vi "水质测量数据table定义.vi"(5 "数据标记表":string(combo)="N", 7 "table 输入":string, 9 "SN":string, 10 "测量模式":T2(ring)=enum."水样测试", 11 "data":T1 {"单位" items=["ug/L", "mg/L", "ppm", "mg/m3", "cm", "ppb", "ug/m3", "%", "nmol/mol", "umol/mol", "MPN/L", "MPN/100ml", "ng/m3", "NTU", "无量纲", "ms/cm", "us/cm"]}) -> (1 "table 输出":string, 2 "columns":string[](array[string]), 3 "data输出":T3)   [LabVIEW 2016, in "挥发酚.lvlib"]
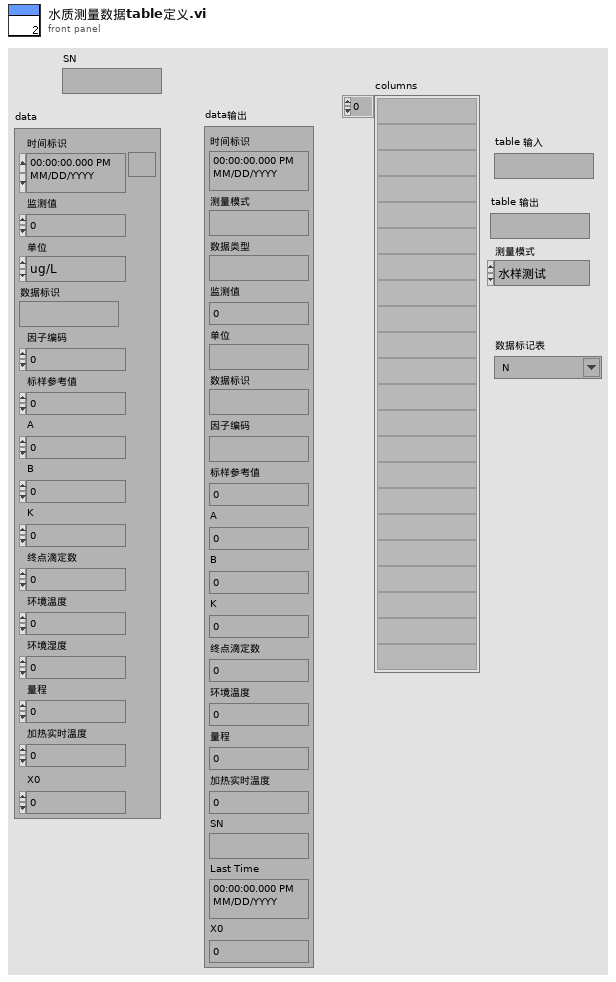
[diagram p1: front panel]
types:
  T1 = cluster{"时间标识":timestamp, "监测值":sgl, "单位":u16, "数据标识":string, "因子编码":u32, "标样参考值":sgl, "A":sgl, "B":sgl, "K":sgl, "终点滴定数":sgl, "环境温度":sgl, "环境湿度":sgl, "量程":sgl, "加热实时温度":sgl, "X0":sgl}
  T2 = enum16{"维护数据", "水样测试", "标样核查", "零点核查", "跨度核查", "空白测试", "平行样测试", "加标回收", "空白校准", "标样校准", "初始化（清洗）"}
  T3 = cluster{"时间标识":timestamp, "测量模式":string, "数据类型":string, "监测值":sgl, "单位":string, "数据标识":string, "因子编码":string, "标样参考值":sgl, "A":sgl, "B":sgl, "K":sgl, "终点滴定数":sgl, "环境温度":sgl, "量程":sgl, "加热实时温度":sgl, "SN":string, "Last Time":timestamp, "X0":sgl}
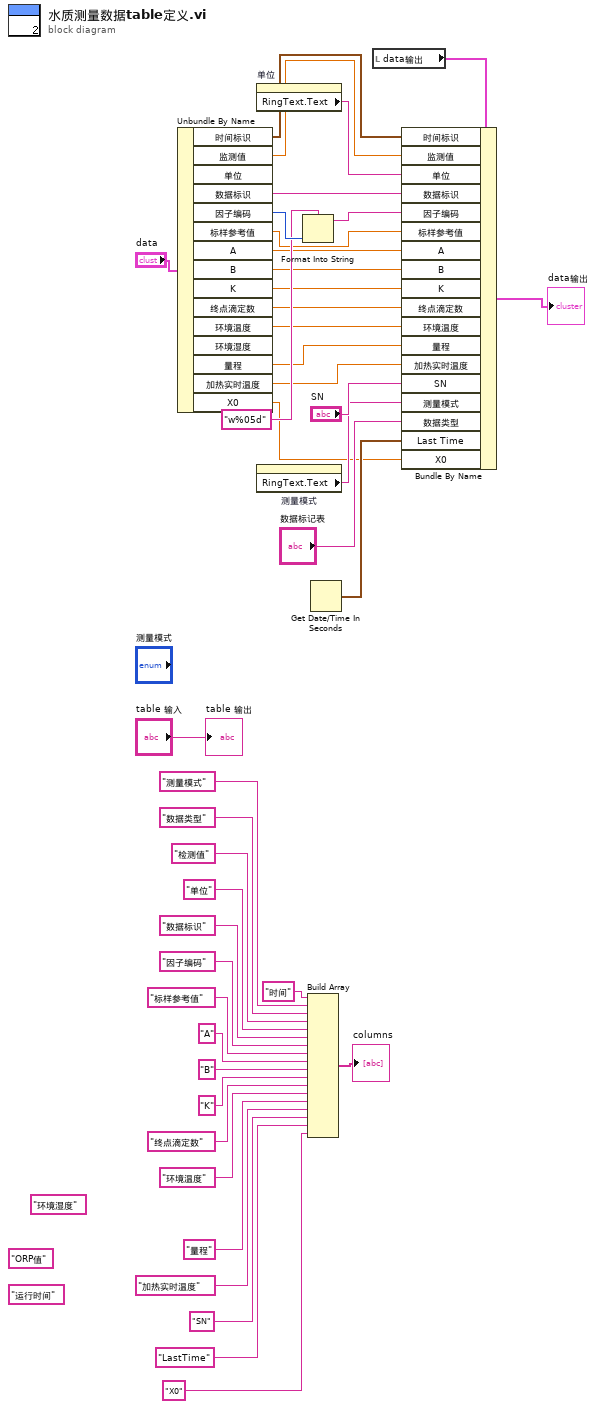
[diagram p0: block diagram]
diagram:
  (unwired) "ORP值"
  (unwired) "环境湿度"
  (unwired) "运行时间"
  n1 = Unbundle By Name("data") -> ("时间标识"=w30:timestamp, "监测值"=w29:sgl, "数据标识"=w28:string, "因子编码"=w33:u32, "标样参考值"=w26:sgl, "A"=w17:sgl, "B"=w16:sgl, "K"=w15:sgl, "终点滴定数"=w14:sgl, "环境温度"=w13:sgl, "量程"=w5:sgl, "加热实时温度"=w12:sgl, "X0"=w2:sgl)  [unwired: 2 out]
  n2 = property on="单位" class="Ring (严格)"() -> ("RingText.Text"=w18:string)  [unwired: 2 in, 2 out]
  n3 = property on="测量模式" class="Enum (严格)"() -> ("RingText.Text"=w10:string)  [unwired: 2 in, 2 out]
  n4 = Format Into String(format string="w%05d" ("格式字符串"), w33) -> (resulting string=w31:string)  [unwired: 2 in, 1 out]
  n5 = Build Array("时间", "测量模式", "数据类型", "检测值", "单位", "数据标识", "因子编码", "标样参考值", "A", "B", "K", "终点滴定数", "环境温度", "量程", "加热实时温度", "SN", "LastTime", "X0") -> (→"columns":string[])
  n6 = Get Date/Time In Seconds() -> (seconds since 1Jan1904=w8:timestamp)
  n7 = local read "data输出"() -> (w4:T3)
  n8 = Bundle By Name(cluster=w4, "时间标识"=w30, "监测值"=w29, "单位"=w18, "数据标识"=w28, "因子编码"=w31, "标样参考值"=w26, "A"=w17, "B"=w16, "K"=w15, "终点滴定数"=w14, "环境温度"=w13, "量程"=w5, "加热实时温度"=w12, "SN"="SN", "测量模式"=w10, "数据类型"="数据标记表", "Last Time"=w8, "X0"=w2) -> (→"data输出":T3)
  "table 输出" <- "table 输入"
